vi "Global_ACT_Data Out.vi"() -> ()   [LabVIEW 2023, in "Pivot FX_ACT.lvlib"]
uses:
  startup.rtexe/Pivot FX_ACT.lvlib
  startup.rtexe/Cluster_HW Output Values.ctl
  startup.rtexe/Cluster_FX_HW All Sensor Values.ctl
  startup.rtexe/Cluster_FX Sensor Values.ctl
  startup.rtexe/Cluster_FX CloseLoop Values.ctl
  startup.rtexe/Cluster_FX Limit Switchs.ctl
  startup.rtexe/Cluster_FX Current Values.ctl
  startup.rtexe/Cluster_FX Output Set Values.ctl
  startup.rtexe/CTRE_Phoenix_MotorControl_ControlMode.ctl
  startup.rtexe/Cluster_SW Output Data.ctl
  ENUM_ACT_State.ctl
panel:
  out "ACT_Template_STATE":T1
  in  "ACT_Template_SW Output":T2
  out "ACT_Template_HW Output":T3 {"Set"."Mode" items=["PercentOutput"=0, "Position"=1, "Velocity"=2, "Current"=3, "Follower"=5, "MotionProfile"=6, "MotionMagic"=7, "MotionProfileArc"=10, "Disabled"=15]}
  in  "ACT_Template_CycleTime(S)":dbl
  # "The Names of the Data items in the Global Variable MUST describe who the Single Writer is\nFor Actuator Globals the the naming convention is\n   \nACT_Lib Name_Data Name\n\nExamples:\nACT_Drive_X axis\nACT_Hopper_AgitatorSpeed"
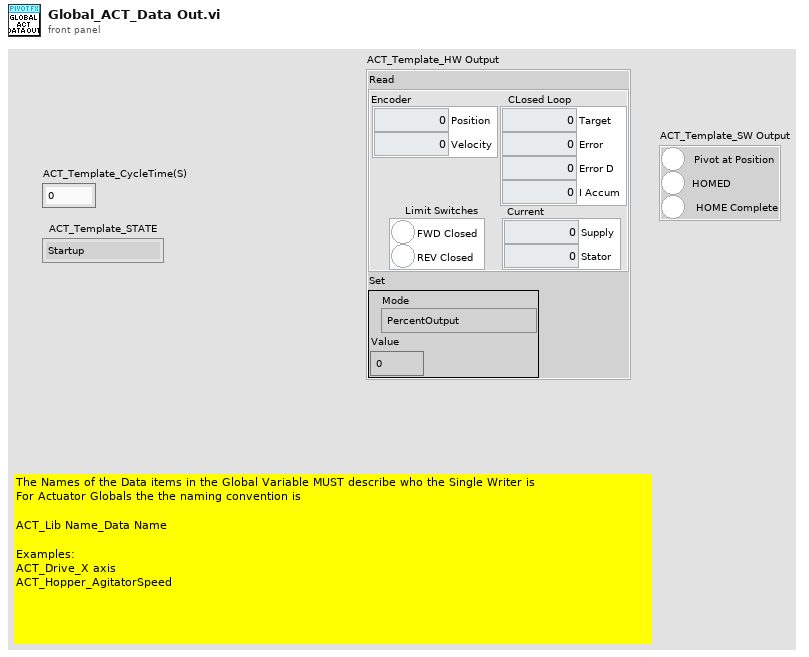
[diagram p1: front panel]
types:
  T1 = typedef "Pivot FX_ACT.lvlib/ENUM_ACT_State.ctl" = enum16{"Startup", "Configuring", "Homming", "Stopping", "Moving Percent Out", "Moving to Position", "Shutdown"}
  T2 = typedef "Pivot FX_ACT.lvlib/Cluster_SW Output Data.ctl" = cluster{"Pivot at Position":bool, "HOMED":bool, "HOME Complete":bool}
  T3 = typedef "Pivot FX_ACT.lvlib/Cluster_HW Output Values.ctl" = cluster{"Read":T4, "Set":T9}
  T4 = typedef "Cluster_FX_HW All Sensor Values.ctl" = cluster{"Encoder":T5, "CLosed Loop":T6, "Limit Switches":T7, "Current":T8}
  T5 = typedef "Cluster_FX Sensor Values.ctl" = cluster{"Position":i32, "Velocity":i32}
  T6 = typedef "Cluster_FX CloseLoop Values.ctl" = cluster{"Target":dbl, "Error":i32, "Error D":dbl, "I Accum":dbl}
  T7 = typedef "Cluster_FX Limit Switchs.ctl" = cluster{"FWD Closed":bool, "REV Closed":bool}
  T8 = typedef "Cluster_FX Current Values.ctl" = cluster{"Supply":dbl, "Stator":dbl}
  T9 = typedef "Cluster_FX Output Set Values.ctl" = cluster{"Mode":T10, "Value":dbl}
  T10 = typedef "CTRE_Phoenix_MotorControl_ControlMode.ctl" = u16
diagram:
